vi "Lock and Save.vi"(8 "error in (no error)":errorcluster, 9 "Revision Comments?":bool, 10 "Lock?":bool, 11 "VI Ref":refnum<vi>) -> (0 "error out":errorcluster, 3 "VI Ref out":refnum<vi>)   [LabVIEW 2014]
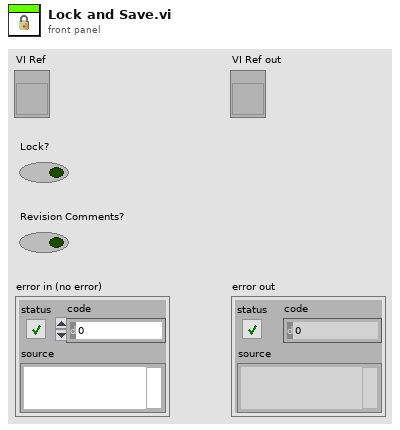
[diagram p1: front panel]
types:
  T1 = enum32{"invalid lock state", "Not Locked", "Locked (No Password)", "Password-protected"}
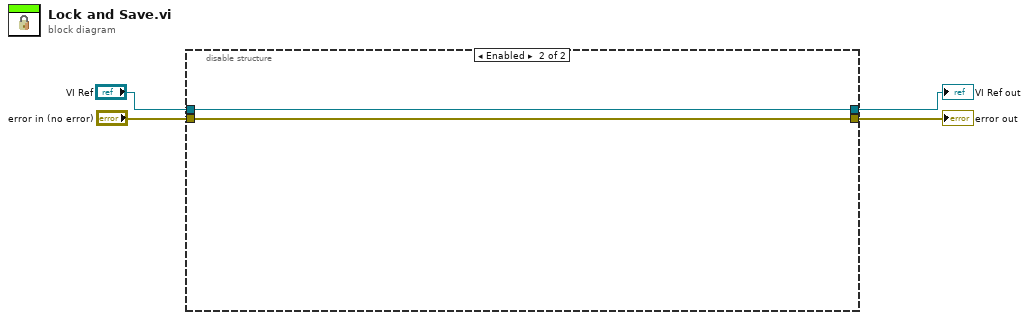
[diagram p0: block diagram]
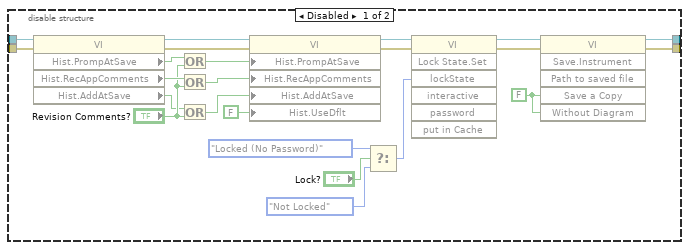
[diagram p2: hidden frame]
diagram:
  n1 = disable-structure shown="Enabled" {
    disable-tunnel: "VI Ref" -> [w27 w29]
    disable-tunnel: "error in (no error)" -> [w26 w28]
    disable-tunnel: [w23 w28] -> w2
    disable-tunnel: [w22 w29] -> w1
    frame Disabled {
      w5 = FALSE ("Save a Copy")
      n2 = property class="VI"(reference=w27, error in=w26) -> (reference out=w17:refnum<vi>, error out=w8:errorcluster, "Hist.PrompAtSave"=w16:bool, "Hist.RecAppComments"=w15:bool, "Hist.AddAtSave"=w13:bool)
      n3 = Or(x=w16, y="Revision Comments?") -> (x .or. y?=w9:bool)
      n4 = Or(x=w15, y="Revision Comments?") -> (x .or. y?=w10:bool)
      n5 = Or(x=w13, y="Revision Comments?") -> (x .or. y?=w11:bool)
      n6 = property class="VI"(reference=w17, error in=w8, "Hist.PrompAtSave"=w9, "Hist.RecAppComments"=w10, "Hist.AddAtSave"=w11, "Hist.UseDflt"=FALSE ("History:Use Defaults")) -> (reference out=w6:refnum<vi>, error out=w7:errorcluster)
      n7 = Select(t=T1."Locked (No Password)" ("Lock State"), s="Lock?", f=T1."Not Locked") -> (s? t:f=w19:T1)
      n8 = invoke class="VI" method="Lock State.Set"(reference=w6, error in=w7, "lockState"=w19) -> (reference out=w25:refnum<vi>, error out=w24:errorcluster)  [unwired: 4 in, 5 out]
      n9 = invoke class="VI" method="Save.Instrument"(reference=w25, error in=w24, "Save a Copy"=w5, "Without Diagram"=w5) -> (reference out=w22:refnum<vi>, error out=w23:errorcluster)  [unwired: 2 in, 4 out]
    }
    frame Enabled {
    }
  }
  "VI Ref out" <- w1
  "error out" <- w2
